vi "GA E Stop Get Sts.vi"(8 "error in (no error)":errorcluster caption="错误输入（无错误）", 11 "nEStopSts":i16) -> (0 "error out":errorcluster caption="错误输出", 2 "function return":i32, 3 "nEStopSts out":i16)   [LabVIEW 2015, in "GAS.lvlib"]
doc: "extern \"C\" __declspec(dllimport) int GA_EStopGetSts(short *nEStopSts);"
uses:
  <userlib>/BP_GAS/GAS.lvlib
  <userlib>/BP_GAS/GAS.dll
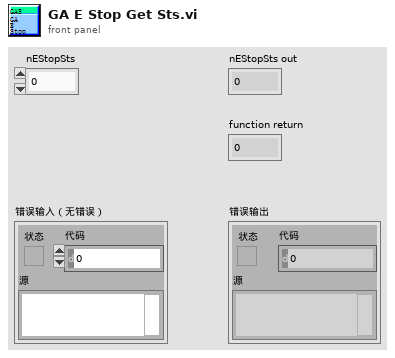
[diagram p1: front panel]
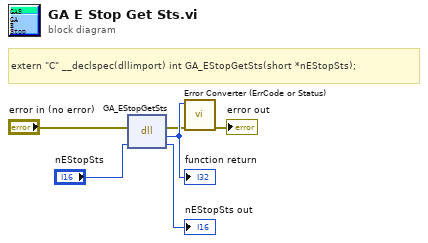
[diagram p0: block diagram]
diagram:
  # "extern \"C\" __declspec(dllimport) int GA_EStopGetSts(short *nEStopSts);"
  n1 = dll-call lib="E:/Program Files (x86)/National Instruments/LabVIEW 2015/user.lib/BP_GAS/GAS.*" fn="GA_EStopGetSts"(error in="error in (no error)", "nEStopSts"="nEStopSts") -> (error out=w2:errorcluster, w6:i32, "nEStopSts"=→"nEStopSts out":i16)  [unwired: 2 in, 1 out]
  "function return" <- w6
  n2 = call "Error Converter (ErrCode or Status).vi"("error in (no error)"=w2, "error code"=w6) -> ("error out"=→"error out":errorcluster)  [unwired: 9 in]
